vi "MoveBySteps.vi"(6 "Direction":enum16{"Forward", "Backwards"}(ring), 7 "Polarity":enum16{"Positive", "Negative"}(ring), 8 "error in (no error)":errorcluster, 9 "Speed":u32, 10 "Steps":u32, 11 "TranslationStage in":refnum<class "ArduinoTranslationStage.lvclass">) -> (0 "error out":errorcluster, 3 "TranslationStage out":refnum<class "ArduinoTranslationStage.lvclass">)   [LabVIEW 2023, in "ArduinoTranslationStage.lvlib" / "ArduinoTranslationStage.lvclass"]
uses:
  ArduinoTranslationStage.lvclass
  <vilib>/Instr/_visa.llb/Select Event Type.ctl
  Interfaces/AbstractInstrumentClasses/TranslationStages_LV/TranslationStagesComm Messages/StageMoveDone Msg/StageMoveDone Msg.lvclass
  <vilib>/ActorFramework/Actor/Actor.lvclass
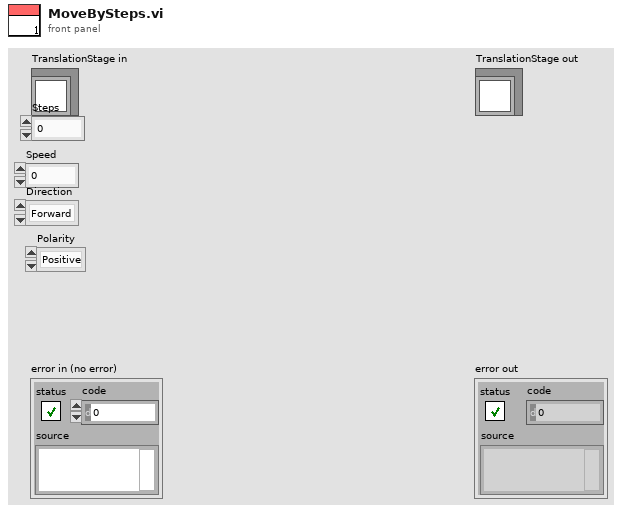
[diagram p1: front panel]
types:
  T1 = typedef "Select Event Type.ctl" = u32
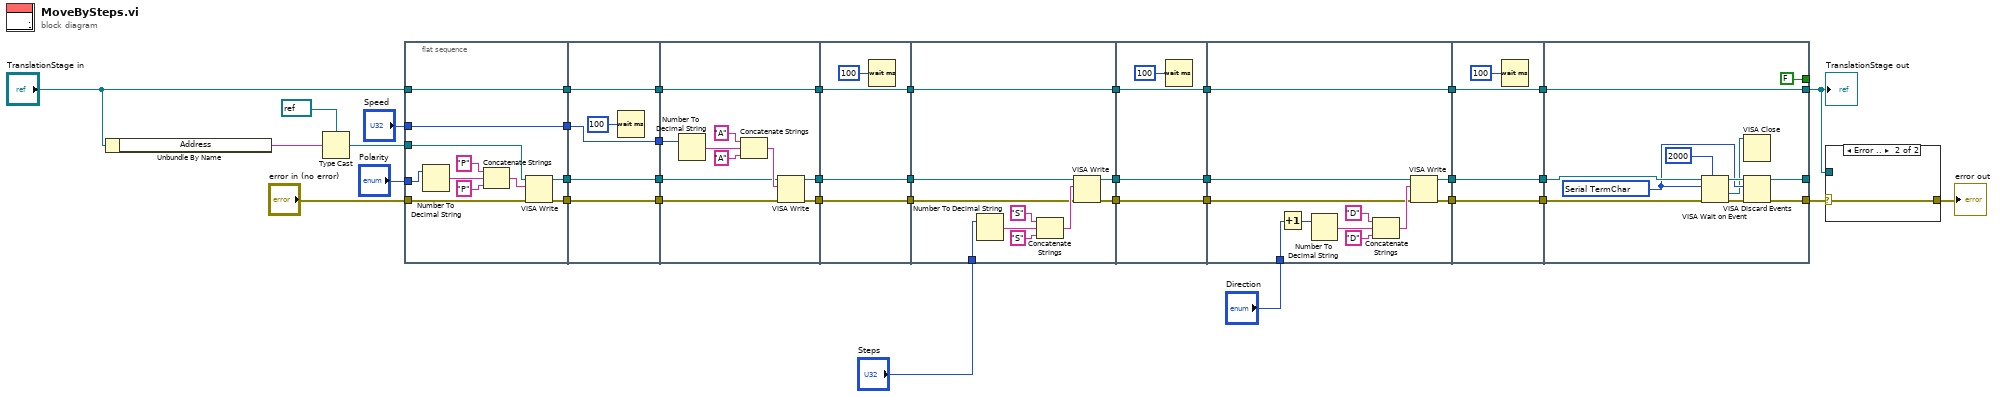
[diagram p0: block diagram]
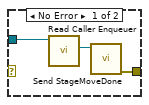
[diagram p2: hidden frame]
diagram:
  n1 = Unbundle By Name("TranslationStage in") -> ("Address"=w16:string)
  n2 = Type Cast(type=refnum<visa-resource-name> refnum ("VISA resource name"), x=w16) -> (*(type *) &x=w15:refnum<visa-resource-name>)
  n3 = flat-sequence {
    tunnel: w15 -> [w41]
    tunnel: "Speed" -> [w49]
    tunnel: "error in (no error)" -> [w45]
    tunnel: [w44] -> w38
    tunnel: [w49] -> w37
    tunnel: [w42] -> w36
    tunnel: "Polarity" -> [w40]
    tunnel: [w39] -> w8
    tunnel: "TranslationStage in" -> [w39]
    tunnel: [w54] -> w35
    tunnel: [w53] -> w34
    tunnel: [w52] -> w33
    tunnel: w38 -> [w54]
    tunnel: w37 -> [w53]
    tunnel: w36 -> [w52]
    tunnel: [w50] -> w9
    tunnel: w8 -> [w50]
    tunnel: [w60] -> w32
    tunnel: [w56] -> w31
    tunnel: w35 -> [w62]
    tunnel: w34 -> [w58]
    tunnel: w33 -> [w57]
    tunnel: [w55] -> w10
    tunnel: w9 -> [w55]
    tunnel: [w67] -> w30
    tunnel: w32 -> [w67]
    tunnel: [w66] -> w29
    tunnel: w31 -> [w66]
    tunnel: [w65] -> w11
    tunnel: w10 -> [w65]
    tunnel: w30 -> [w75]
    tunnel: [w74] -> w27
    tunnel: [w72] -> w28
    tunnel: "Steps" -> [w71]
    tunnel: w29 -> [w70]
    tunnel: [w69] -> w12
    tunnel: w11 -> [w69]
    tunnel: [w82] -> w26
    tunnel: [w81] -> w25
    tunnel: w28 -> [w81]
    tunnel: w27 -> [w82]
    tunnel: [w79] -> w13
    tunnel: w12 -> [w79]
    tunnel: [w93] -> w24
    tunnel: [w92] -> w23
    tunnel: w26 -> [w85]
    tunnel: w25 -> [w86]
    tunnel: "Direction" -> [w84]
    tunnel: [w83] -> w14
    tunnel: w13 -> [w83]
    tunnel: w24 -> [w97]
    tunnel: w23 -> [w96]
    tunnel: [w97] -> w21
    tunnel: [w96] -> w22
    tunnel: w14 -> [w94]
    tunnel: [w94] -> w6
    tunnel: w22 -> [w107]
    tunnel: w21 -> [w99]
    tunnel: [w103] -> _
    tunnel: [w102] -> w4
    tunnel: [FALSE ("event data")] -> _
    tunnel: [w100] -> w5
    tunnel: w6 -> [w100]
    frame #0 {
      n4 = Number To Decimal String(number=w40) -> (decimal integer string=w46:string)  [unwired: 1 in]
      n5 = Concatenate Strings("P" ("write buffer"), w46, "P" ("string")) -> (w47:string)
      n6 = VISA Write(VISA resource name=w41, write buffer=w47, error in (no error)=w45) -> (VISA resource name out=w42:refnum<visa-resource-name>, error out=w44:errorcluster)  [unwired: 1 out]
    }
    frame #1 {
      n7 = Wait (ms)(milliseconds to wait=u32 100) -> ()  [unwired: 1 out]
    }
    frame #2 {
      n8 = Number To Decimal String(number=w58) -> (decimal integer string=w59:string)  [unwired: 1 in]
      n9 = Concatenate Strings("A" ("write buffer"), w59, "A" ("string")) -> (w61:string)
      n10 = VISA Write(VISA resource name=w57, write buffer=w61, error in (no error)=w62) -> (VISA resource name out=w56:refnum<visa-resource-name>, error out=w60:errorcluster)  [unwired: 1 out]
    }
    frame #3 {
      n11 = Wait (ms)(milliseconds to wait=u32 100) -> ()  [unwired: 1 out]
    }
    frame #4 {
      n12 = Number To Decimal String(number=w71) -> (decimal integer string=w73:string)  [unwired: 1 in]
      n13 = Concatenate Strings("S" ("write buffer"), w73, "S" ("string")) -> (w76:string)
      n14 = VISA Write(VISA resource name=w70, write buffer=w76, error in (no error)=w75) -> (VISA resource name out=w72:refnum<visa-resource-name>, error out=w74:errorcluster)  [unwired: 1 out]
    }
    frame #5 {
      n15 = Wait (ms)(milliseconds to wait=u32 100) -> ()  [unwired: 1 out]
    }
    frame #6 {
      n16 = Increment(x=w84) -> (x+1=w88:enum16{"Forward", "Backwards"})
      n17 = Number To Decimal String(number=w88) -> (decimal integer string=w87:string)  [unwired: 1 in]
      n18 = Concatenate Strings("D" ("write buffer"), w87, "D" ("string")) -> (w90:string)
      n19 = VISA Write(VISA resource name=w86, write buffer=w90, error in (no error)=w85) -> (VISA resource name out=w92:refnum<visa-resource-name>, error out=w93:errorcluster)  [unwired: 1 out]
    }
    frame #7 {
      n20 = Wait (ms)(milliseconds to wait=u32 100) -> ()  [unwired: 1 out]
    }
    frame #8 {
      w104 = T1 1073684516 items=["Service Request"=1073684491, "Trigger"=3221168138, "Clear"=1073684493, "VXI Signal"=1073684512, "VXI/VME Interrupt"=3221168161, "VXI/VME Sysfail"=1073684509, "VXI/VME Sysreset"=1073684510, "GPIB CIC"=1073684498, "GPIB Talk"=1073684499, "GPIB Listen"=1073684500, "PXI Interrupt"=1073684514, "Serial Break"=1073684515, "Serial TermChar"=1073684516, "Serial CTS"=1073684521, "Serial DSR"=1073684522, "Serial DCD"=1073684524, "Serial RI"=1073684526, "Serial Character"=1073684533, "USB Interrupt"=1073684535, "All Enabled"=1073709055] ("Event Type")
      n21 = VISA Wait on Event(7:u32 2000 ("timeout (0)"), 8:w99, 10:w104, 11:w107) -> (0:w105:errorcluster, 1:w98:refnum<visa-resource-name>, 3:w106:refnum<visa-resource-name>)  [unwired: 1 in, 1 out]
      n22 = VISA Close(VISA resource name=w98) -> ()  [unwired: 1 in, 1 out]
      n23 = VISA Discard Events(8:w105, 10:w104, 11:w106) -> (0:w102:errorcluster, 3:w103:refnum<visa-resource-name>)  [unwired: 1 in]
    }
  }
  n24 = case shown="Error .." w4 {
    selector: w4 -> [_ w112]
    tunnel: [w111 w112] -> w3
    tunnel: w5 -> [w109 _]
    frame No Error {
      n25 = call <vilib>:"Read Caller Enqueuer.vi"("Actor"=w109) -> ("Caller Enqueuer"=w110:refnum<class "Message Enqueuer.lvclass">)  [unwired: 10 in]
      n26 = call "Send StageMoveDone.vi"("Message Enqueuer"=w110) -> ("error out"=w111:errorcluster)  [unwired: 9 in, 1 out]
    }
    frame Error {
    }
  }
  "error out" <- w3
  "TranslationStage out" <- w5
